vi "Teleop.vi"(10 "Match Info":T2={"Autonomous Elapsed Seconds"=0.0, "TeleOp Elapsed Seconds"=0.0, "Disabled Elapsed Seconds"=0.0, "Visited Autonomous"=FALSE, "Visited TeleOp"=FALSE, "Visited Disabled"=FALSE, "Autonomous Settings"={"Autonomous Style"=enum."Independent", "VI Refnum"=refnum}}, 11 "Call Context":T3) -> ()   [LabVIEW 2015]
doc: "This VI is called for each TeleOp packet received from the DS where the robot is not disabled. It is often used to read from the joysticks and update I/O or to update setpoints for timed control loops. It should complete and return within 20 milliseconds or it may miss DS packets."
uses:
  <vilib>/Rock Robotics/WPI/DriverStation/WPI_DriverStationDerivedRobotMode.ctl
  <vilib>/Rock Robotics/WPI/DriverStation/WPI_DriverStationMatch Info.ctl
  <vilib>/Rock Robotics/WPI/Utilities/WPI_GetSetVariantRefNum.vi
  <vilib>/Rock Robotics/Network Tables/NT Write Boolean Array.vi
  <vilib>/Rock Robotics/Network Tables/NT Write Numeric Array.vi
  <vilib>/Rock Robotics/Network Tables/NT Read Boolean.vi
  <vilib>/Rock Robotics/Network Tables/NT Read Number.vi
  Robot Global Data.vi
  <vilib>/Rock Robotics/Network Tables/NT Write Number.vi
  <vilib>/Rock Robotics/WPI/RobotDrive/WPI_RobotDriveArcadeDrive_Standard(NoSaturation).vi
panel:
  in  "Winch Lock":bool
  out "Ladder Up Start Time":u32
  in  "LadderStateMachine":i32
  out "Accelerations":T1
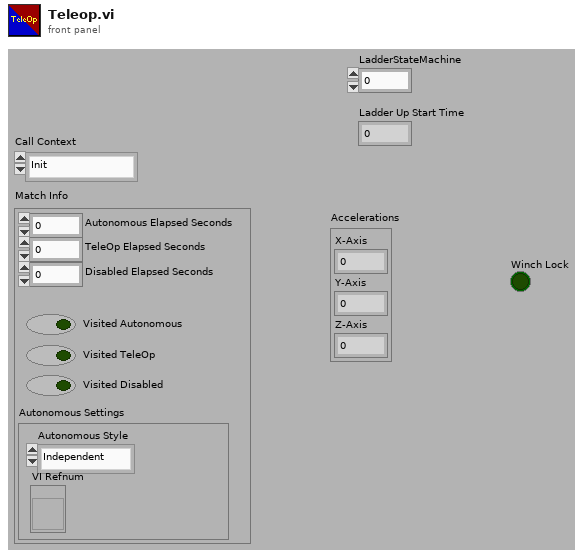
[diagram p1: front panel]
types:
  T1 = cluster{"X-Axis":dbl, "Y-Axis":dbl, "Z-Axis":dbl}
  T2 = typedef "WPI_DriverStationMatch Info.ctl" = cluster{"Autonomous Elapsed Seconds":dbl, "TeleOp Elapsed Seconds":dbl, "Disabled Elapsed Seconds":dbl, "Visited Autonomous":bool, "Visited TeleOp":bool, "Visited Disabled":bool, "Autonomous Settings":cluster{"Autonomous Style":enum16{"Iterative", "Independent"}, "VI Refnum":refnum<vi>}}
  T3 = typedef "WPI_DriverStationDerivedRobotMode.ctl" = enum16{"Init", "Execute", "Stop"}
  T4 = typedef "WPI_RobotDriveDevRef.ctl" = cluster{"DevStatus":errorcluster, "Motors[]":T5[], "Square Inputs":bool, "Max Output":dbl}
  T5 = typedef "WPI_MotorControlDeviceRef.ctl" = cluster{"DeviceStatus":errorcluster, "Type":T6, "PWM":cluster{"PWM Channel":T7, "DeadBand":T8}, "CAN":cluster{"Device Number":u8, "Control Mode":T9, "Semaphore":T10, "Max Vout":dbl, "TalonSRX Control Mode":T11}, "Invert":bool}
  T6 = typedef "WPI_MotorControlType.ctl" = enum16{"PWM", "CAN", "CANTalonSRX"}
  T7 = typedef "FPGA_DIOPWMChannel.ctl" = enum8{"PWM 0", "PWM 1", "PWM 2", "PWM 3", "PWM 4", "PWM 5", "PWM 6", "PWM 7", "PWM 8", "PWM 9", "PWM MXP 0", "PWM MXP 1", "PWM MXP 2", "PWM MXP 3", "PWM MXP 4", "PWM MXP 5", "PWM MXP 6", "PWM MXP 7", "PWM MXP 8", "PWM MXP 9", "Invalid"}
  T8 = typedef "WPI_PWMDeadband.ctl" = cluster{"Name":string, "maxPositivePwm":i32, "minPositivePwm":i32, "centerPwm":i32, "maxNegativePwm":i32, "minNegativePwm":i32, "angularRange":u16}
  T9 = typedef "WPI_CANJaguar_ControlMode.ctl" = enum8{"Percent VBus", "Current", "Speed", "Position", "Voltage"}
  T10 = typedef "Semaphore RefNum" = refnum<k1>
  T11 = typedef "WPI_CANTalonSRX_APIControlMode.ctl" = enum8{"Percent VBus", "Speed", "Position", "Slave", "Unchanged / Invalid", "Voltage Compensation", "Current", "Motion Profile"}
  T12 = typedef "WPI_JoystickDevRef.ctl" = cluster{"Device":T13}
  T13 = typedef "WPI_JoystickDeviceEnum.ctl" = enum16{"USB 0", "USB 1", "USB 2", "USB 3", "USB 4", "USB 5"}
  T14 = typedef "WPI_DigitalInputDevRef.ctl" = cluster{"DevStatus":errorcluster, "DIO Channel":T15}
  T15 = typedef "FPGA_DIOChannel.ctl" = enum8{"DIO 0", "DIO 1", "DIO 2", "DIO 3", "DIO 4", "DIO 5", "DIO 6", "DIO 7", "DIO 8", "DIO 9", "DIO MXP 0", "DIO MXP 1", "DIO MXP 2", "DIO MXP 3", "DIO MXP 4", "DIO MXP 5", "DIO MXP 6", "DIO MXP 7", "DIO MXP 8", "DIO MXP 9", "DIO MXP 10", "DIO MXP 11", "DIO MXP 12", "DIO MXP 13", "DIO MXP 14", "DIO MXP 15", "Invalid"}
  T16 = typedef "WPI_AccelerometerDevRef.ctl" = cluster{"DevStatus":errorcluster, "Scaling":T17, "Analog Channels":T18, "I2C Bus":T20, "SPI Bus":T21, "Accel Range":T22, "ADXL Axes":T23, "Handle":i32, "Device Address":u8, "Accel Type":enum16{"Analog", "ADXL345 I2C", "ADXL345 SPI", "Internal", "ADXL362 SPI"}}
  T17 = typedef "WPI_AccelerometerScaling.ctl" = cluster{"Gain (VoltsPerG)":dbl, "Center Voltage":dbl}
  T18 = typedef "WPI_AccelerometerAnalogChannels.ctl" = cluster{"X-Axis":T19, "Y-Axis":T19, "Z-Axis":T19}
  T19 = typedef "FPGA_AIChannel.ctl" = enum8{"AI 0", "AI 1", "AI 2", "AI 3", "AI MXP 0", "AI MXP 1", "AI MXP 2", "AI MXP 3", "Invalid"}
  T20 = typedef "i2c_bus.ctl" = enum16{"I2C On-Board", "I2C MXP", "Invalid"}
  T21 = typedef "spi_bus.ctl" = enum16{"SPI On-Board, CS0", "SPI On-Board, CS1", "SPI On-Board, CS2", "SPI On-Board, CS3", "SPI MXP", "Invalid"}
  T22 = typedef "ADXL345 Range.ctl" = u8
  T23 = typedef "WPI_AccelerometerADXL345 Axes.ctl" = cluster{"X-Axis":bool, "Y-Axis":bool, "Z-Axis":bool}
  T24 = typedef "WPI_EncoderDevRef.ctl" = cluster{"DevStatus":errorcluster, "EncoderIndex":T25, "CounterIndex":T26, "DistancePerCount":dbl, "Decoding Type":T27}
  T25 = typedef "FPGA_EncoderIdx.ctl" = enum8{"Enc 0", "Enc 1", "Enc 2", "Enc 3", "Enc 4", "Enc 5", "Enc 6", "Enc 7", "Invalid"}
  T26 = typedef "FPGA_CounterCtrSystemIndex.ctl" = enum8{"Ctr 0", "Ctr 1", "Ctr 2", "Ctr 3", "Ctr 4", "Ctr 5", "Ctr 6", "Ctr 7", "Invalid"}
  T27 = typedef "WPI_EncoderType.ctl" = enum16{"1x", "2x", "4x"}
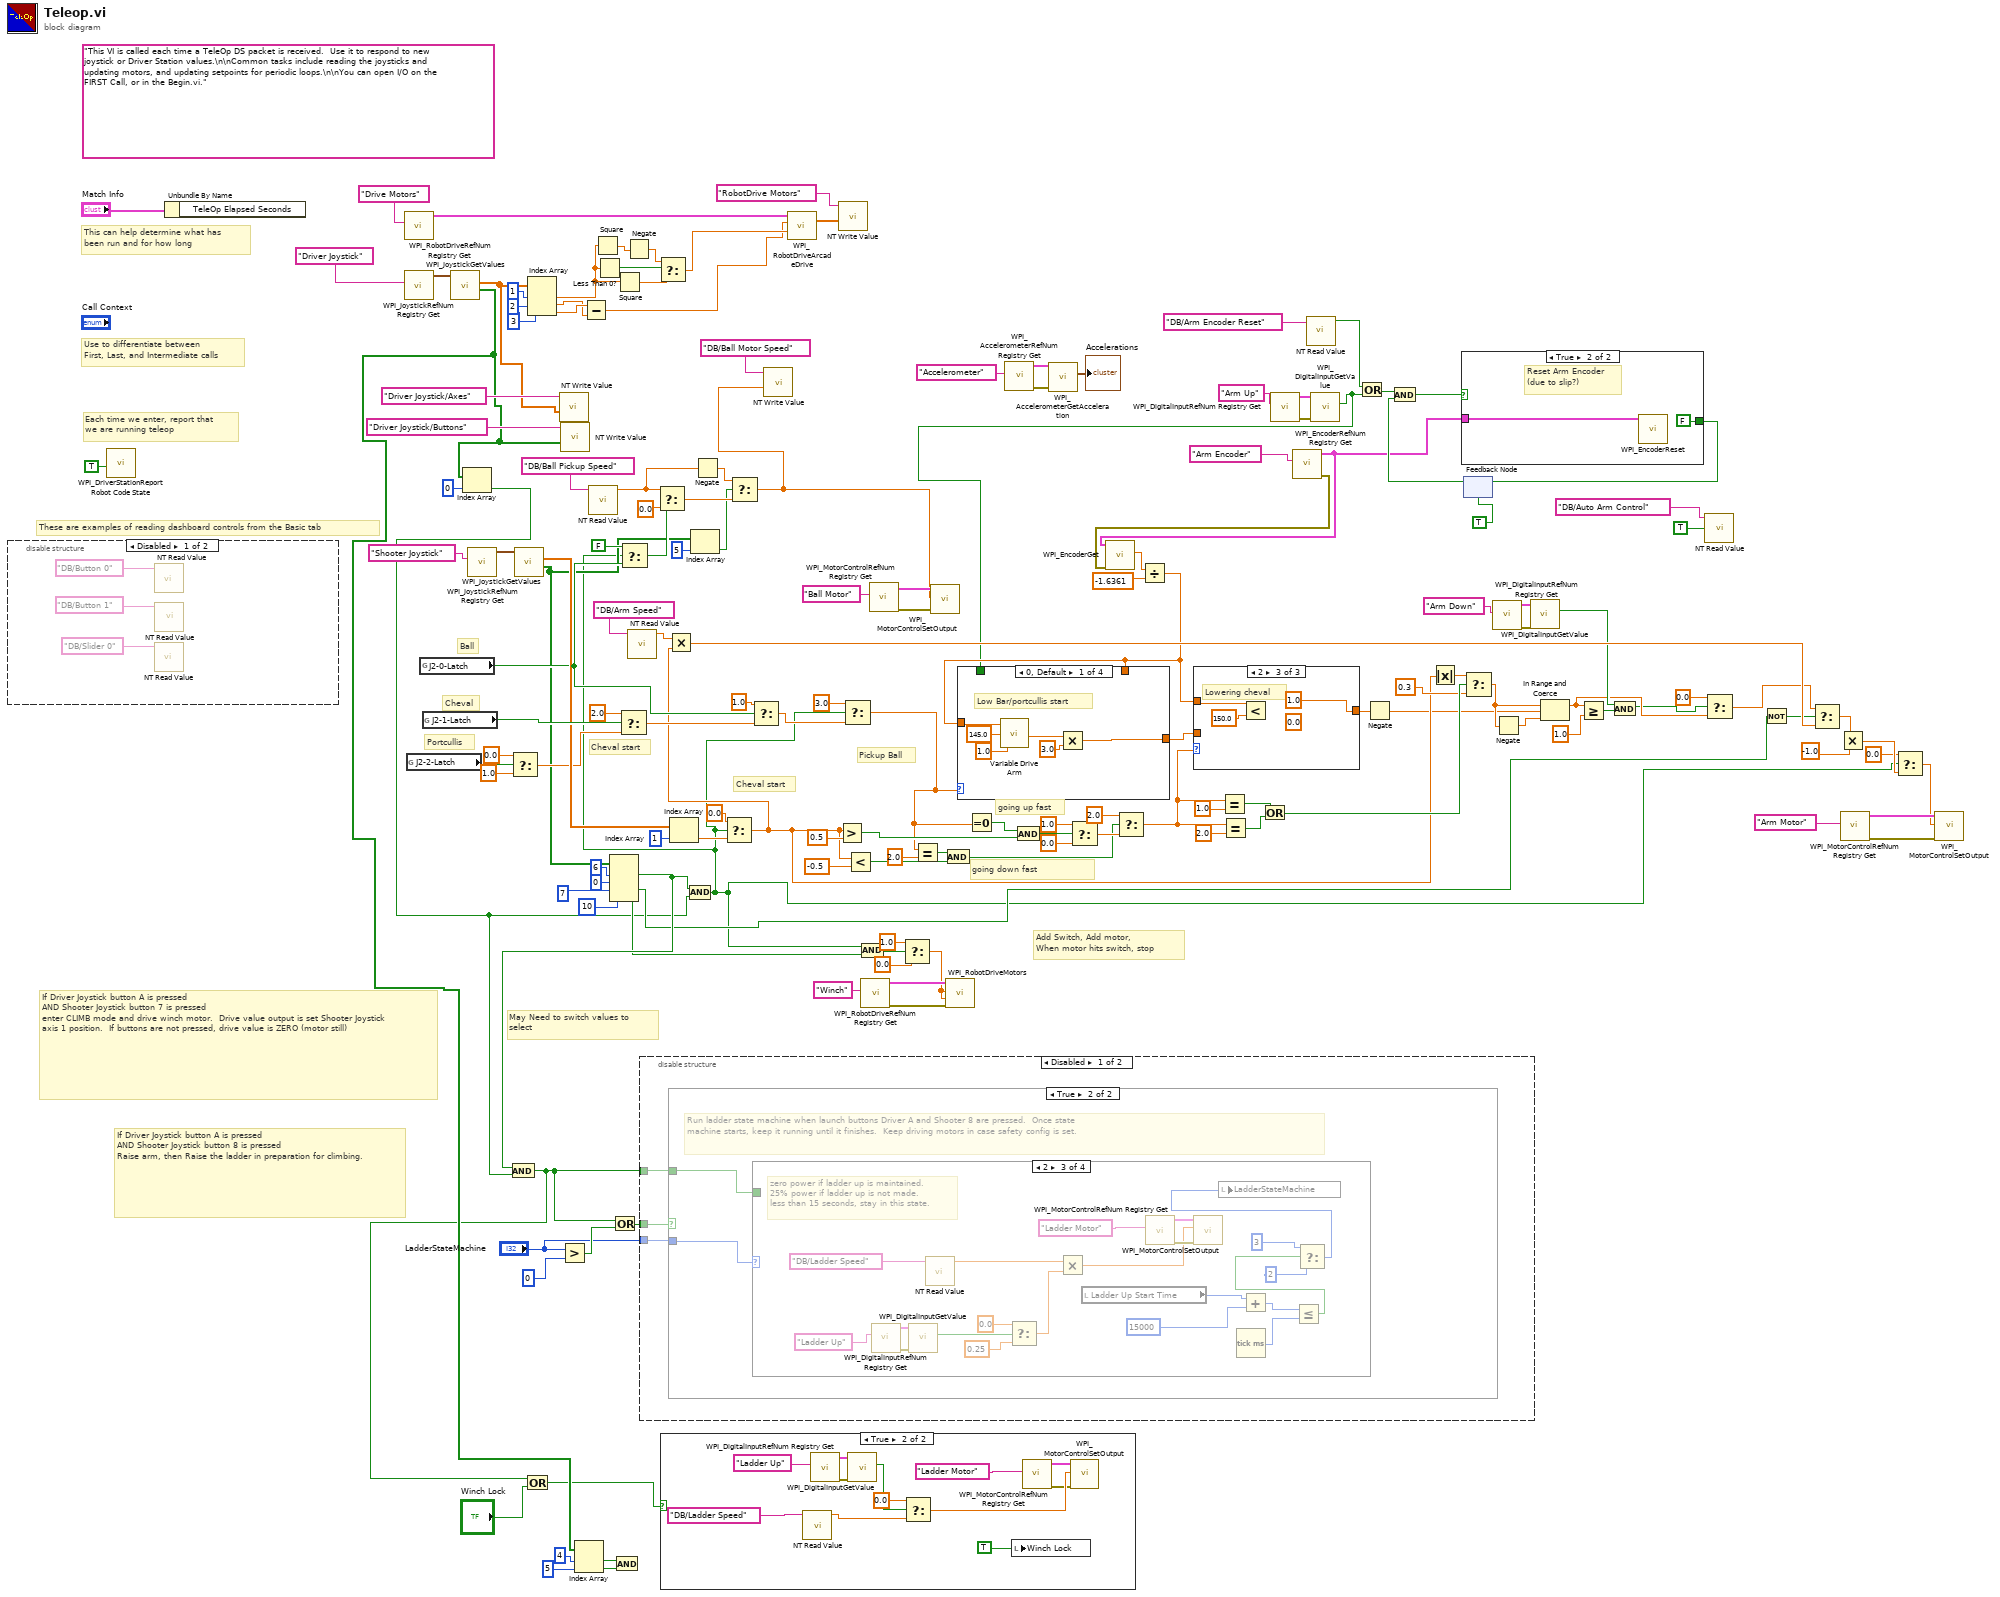
[diagram p0: block diagram]
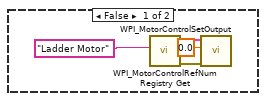
[diagram p2: hidden frame]
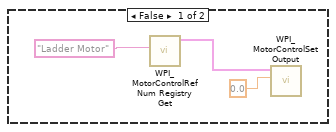
[diagram p3: hidden frame]
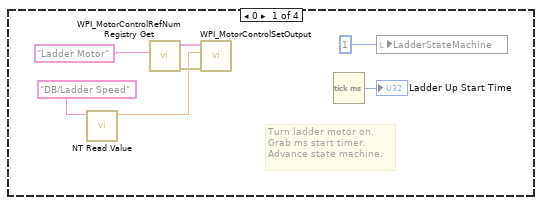
[diagram p4: hidden frame]
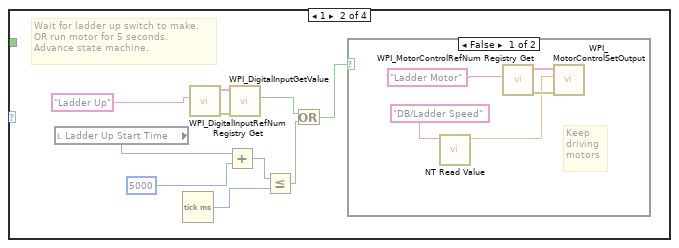
[diagram p5: hidden frame]
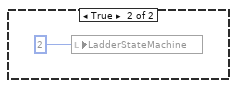
[diagram p6: hidden frame]
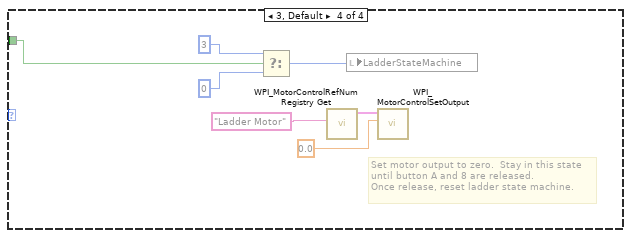
[diagram p7: hidden frame]
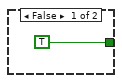
[diagram p9: hidden frame]
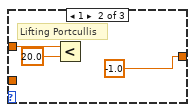
[diagram p12: hidden frame]
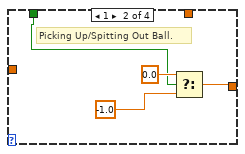
[diagram p13: hidden frame]
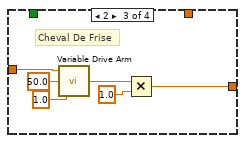
[diagram p14: hidden frame]
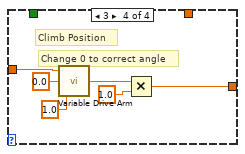
[diagram p15: hidden frame]
diagram:
  (unwired) "This VI is called each time a TeleOp DS packet is received.  Use it to respond to new joystick or Driver Station values.\n\nCommon tasks include reading the joysticks and updating motors, and updating setpoints for periodic loops.\n\nYou can open I/O on the FIRST Call, or in the Begin.vi."
  # "going up fast"
  # "going down fast"
  # "If Driver Joystick button A is pressed\nAND Shooter Joystick button 8 is pressed\nRaise arm, then Raise the ladder in preparation for climbing."
  # "If Driver Joystick button A is pressed\nAND Shooter Joystick button 7 is pressed\nenter CLIMB mode and drive winch motor.  Drive value output is set Shooter Joystick axis 1 position.  If buttons are not pressed, drive value is ZERO (motor still)"
  # "Add Switch, Add motor, \nWhen motor hits switch, stop"
  # "Portcullis"
  # "Ball"
  # "Cheval"
  # "May Need to switch values to \nselect"
  # "Cheval start"
  # "Pickup Ball"
  # "Cheval start"
  # "These are examples of reading dashboard controls from the Basic tab"
  # "Each time we enter, report that\nwe are running teleop"
  # "Use to differentiate between\nFirst, Last, and Intermediate calls"
  # "This can help determine what has\nbeen run and for how long"
  n1 = disable-structure shown="Disabled" {
    frame Disabled {
      n2 = call-poly <vilib>:"NT Read Value.vi"("Name"="DB/Button 0" ("refnum name")) -> ("Boolean"=w158:bool)  [unwired: 9 in, 1 out]
      n3 = call-poly <vilib>:"NT Read Value.vi"("Name"="DB/Slider 0" ("refnum name")) -> ("Numeric"=w160:dbl)  [unwired: 9 in, 1 out]
      n4 = call-poly <vilib>:"NT Read Value.vi"("Name"="DB/Button 1" ("refnum name")) -> ("Boolean"=w159:bool)  [unwired: 9 in, 1 out]
    }
    frame Enabled {
    }
  }
  n5 = call <vilib>:"WPI_DriverStationReport Robot Code State.vi"("TeleOp"=TRUE ("Autonomous")) -> ()  [unwired: 10 in, 1 out]
  n6 = Unbundle By Name("Match Info") -> ()  [unwired: 1 out]
  n7 = call <vilib>:"WPI_RobotDriveRefNum Registry Get.vi"("refnum name"="Drive Motors") -> ("RobotDriveDevRef"=w154:T4)  [unwired: 1 in, 9 out]
  n8 = call <vilib>:"WPI_JoystickRefNum Registry Get.vi"("refnum name"="Driver Joystick") -> ("JoystickDevRef"=w152:T12)  [unwired: 1 in, 9 out]
  n9 = global read "Robot Global Data.vi" "J2-2-Latch"() -> (w77:bool)
  n10 = global read "Robot Global Data.vi" "J2-0-Latch"() -> (w73:bool)
  n11 = global read "Robot Global Data.vi" "J2-1-Latch"() -> (w130:bool)
  n12 = call <vilib>:"WPI_JoystickGetValues.vi"("JoystickDevRef"=w152) -> ("Buttons"=w20:bool[], "Axes"=w142:dbl[])  [unwired: 6 in, 3 out]
  n13 = Index Array(array=w20, index=0) -> (element=w19:bool)
  n14 = call <vilib>:"WPI_JoystickRefNum Registry Get.vi"("refnum name"="Shooter Joystick") -> ("JoystickDevRef"=w141:T12)  [unwired: 1 in, 9 out]
  n15 = Select(t=0.0, s=w77, f=1.0) -> (s? t:f=w78:dbl)
  n16 = call <vilib>:"WPI_JoystickGetValues.vi"("JoystickDevRef"=w141) -> ("Buttons"=w44:bool[], "Axes"=w106:dbl[])  [unwired: 6 in, 3 out]
  n17 = Index Array(array=w142, index #1=1 ("index"), index #2=2 ("index"), index #3=3 ("index")) -> (element #1=w102:dbl, element #2=w99:dbl, element #3=w100:dbl)
  n18 = call-poly <vilib>:"NT Write Value.vi"("Numeric Array"=w142, "Name"="Driver Joystick/Axes") -> ()  [unwired: 9 in, 1 out]
  n19 = call-poly <vilib>:"NT Write Value.vi"("Boolean Array"=w20, "Name"="Driver Joystick/Buttons") -> ()  [unwired: 9 in, 1 out]
  n20 = Greater?(x="LadderStateMachine", y=0) -> (0:w58:bool)
  n21 = Index Array(array=w20, index #1=4 ("index"), index #2=5 ("index")) -> (element #1=w15:bool, element #2=w16:bool)
  n22 = Subtract(x=w100, y=w99) -> (x-y=w98:dbl)
  n23 = call-poly <vilib>:"NT Read Value.vi"("Name"="DB/Ball Pickup Speed") -> ("Numeric"=w45:dbl)  [unwired: 9 in, 1 out]
  n24 = Square(x=w102) -> (x^2=w146:dbl)
  n25 = Less Than 0?(x=w102) -> (x < 0?=w148:bool)
  n26 = Index Array(array=w44, index #1=6 ("index"), index #2=0 ("index"), index #3=7 ("index"), index #4=10 ("index")) -> (element #1=w55:bool, element #3=w36:bool, element #4=w24:bool)  [unwired: 1 out]
  n27 = And(x=w55, y=w19) -> (x .and. y?=w13:bool)
  n28 = Or(x=w13, y="Winch Lock") -> (x .or. y?=w2:bool)
  n29 = Or(x=w13, y=w58) -> (x .or. y?=w57:bool)
  n30 = And(x=w15, y=w16) -> ()  [unwired: 1 out]
  n31 = Square(x=w102) -> (x^2=w145:dbl)
  n32 = Select(t=2.0, s=w130, f=w78) -> (s? t:f=w131:dbl)
  n33 = Negate(x=w146) -> (-x=w147:dbl)
  n34 = call-poly <vilib>:"NT Read Value.vi"("Name"="DB/Arm Speed") -> ("Numeric"=w67:dbl)  [unwired: 9 in, 1 out]
  n35 = disable-structure shown="Disabled" {
    disable-tunnel: w57 -> [w166 _]
    disable-tunnel: "LadderStateMachine" -> [w165 _]
    disable-tunnel: w13 -> [w164 _]
    frame Disabled {
      n36 = case shown="True" w166 {
        tunnel: w165 -> [_ w171]
        tunnel: w164 -> [_ w170]
        frame False {
          n37 = call <vilib>:"WPI_MotorControlRefNum Registry Get.vi"("refnum name"="Ladder Motor") -> ("MotorControlDevRef"=w167:T5)  [unwired: 9 in, 1 out]
          n38 = call <vilib>:"WPI_MotorControlSetOutput.vi"("Output"=0.0, "MotorControlDevRef"=w167) -> ()  [unwired: 7 in, 3 out]
        }
        frame True {
          # "Run ladder state machine when launch buttons Driver A and Shooter 8 are pressed.  Once state\nmachine starts, keep it running until it finishes.  Keep driving motors in case safety config is set."
          n39 = case shown="2" w171 {
            tunnel: w170 -> [_ _ _ w220]
            frame 0 {
              # "Turn ladder motor on.\nGrab ms start timer.\nAdvance state machine."
              n40 = call-poly <vilib>:"NT Read Value.vi"("Name"="DB/Ladder Speed") -> ("Numeric"=w174:dbl)  [unwired: 9 in, 1 out]
              n41 = call <vilib>:"WPI_MotorControlRefNum Registry Get.vi"("refnum name"="Ladder Motor") -> ("error out"=w178:errorcluster, "MotorControlDevRef"=w177:T5)  [unwired: 9 in]
              n42 = call <vilib>:"WPI_MotorControlSetOutput.vi"("error in (no error)"=w178, "Output"=w174, "MotorControlDevRef"=w177) -> ()  [unwired: 6 in, 3 out]
              n43 = Tick Count (ms)() -> (millisecond timer value=→"Ladder Up Start Time":u32)
              n44 = local write "LadderStateMachine"(1 ("LadderStateMachine")) -> ()
            }
            frame 1 {
              # "Wait for ladder up switch to make.\nOR run motor for 5 seconds.\nAdvance state machine."
              n45 = local read "Ladder Up Start Time"() -> (w184:u32)
              n46 = Tick Count (ms)() -> (millisecond timer value=w182:u32)
              n47 = call <vilib>:"WPI_DigitalInputRefNum Registry Get.vi"("refnum name"="Ladder Up") -> ("error out"=w188:errorcluster, "DigitalInputDevRef"=w186:T14)  [unwired: 9 in]
              n48 = Add(x=w184, y=u32 5000) -> (x+y=w183:u32)
              n49 = call <vilib>:"WPI_DigitalInputGetValue.vi"("error in (no error)"=w188, "DigitalInputDevRef"=w186) -> ("Value"=w179:bool)  [unwired: 7 in, 2 out]
              n50 = Less Or Equal?(x=w183, y=w182) -> (x <= y?=w180:bool)
              n51 = Or(x=w179, y=w180) -> (x .or. y?=w181:bool)
              n52 = case shown="False" w181 {
                frame False {
                  # "Keep\ndriving \nmotors"
                  n53 = call-poly <vilib>:"NT Read Value.vi"("Name"="DB/Ladder Speed") -> ("Numeric"=w189:dbl)  [unwired: 9 in, 1 out]
                  n54 = call <vilib>:"WPI_MotorControlRefNum Registry Get.vi"("refnum name"="Ladder Motor") -> ("error out"=w193:errorcluster, "MotorControlDevRef"=w192:T5)  [unwired: 9 in]
                  n55 = call <vilib>:"WPI_MotorControlSetOutput.vi"("error in (no error)"=w193, "Output"=w189, "MotorControlDevRef"=w192) -> ()  [unwired: 6 in, 3 out]
                }
                frame True {
                  n56 = local write "LadderStateMachine"(2 ("LadderStateMachine")) -> ()
                }
              }
            }
            frame 2 {
              # "zero power if ladder up is maintained.\n25% power if ladder up is not made.\nless than 15 seconds, stay in this state."
              n57 = call <vilib>:"WPI_DigitalInputRefNum Registry Get.vi"("refnum name"="Ladder Up") -> ("error out"=w209:errorcluster, "DigitalInputDevRef"=w207:T14)  [unwired: 9 in]
              n58 = call <vilib>:"WPI_DigitalInputGetValue.vi"("error in (no error)"=w209, "DigitalInputDevRef"=w207) -> ("Value"=w206:bool)  [unwired: 7 in, 2 out]
              n59 = call-poly <vilib>:"NT Read Value.vi"("Name"="DB/Ladder Speed") -> ("Numeric"=w211:dbl)  [unwired: 9 in, 1 out]
              n60 = Select(t=0.0, s=w206, f=0.25 ("y")) -> (s? t:f=w203:dbl)
              n61 = Multiply(x=w211, y=w203) -> (x*y=w210:dbl)
              n62 = local read "Ladder Up Start Time"() -> (w201:u32)
              n63 = call <vilib>:"WPI_MotorControlRefNum Registry Get.vi"("refnum name"="Ladder Motor") -> ("error out"=w215:errorcluster, "MotorControlDevRef"=w214:T5)  [unwired: 9 in]
              n64 = call <vilib>:"WPI_MotorControlSetOutput.vi"("error in (no error)"=w215, "Output"=w210, "MotorControlDevRef"=w214) -> ()  [unwired: 6 in, 3 out]
              n65 = Tick Count (ms)() -> (millisecond timer value=w199:u32)
              n66 = Add(x=w201, y=u32 15000) -> (x+y=w200:u32)
              n67 = Less Or Equal?(x=w200, y=w199) -> (x <= y?=w198:bool)
              n68 = Select(t=3 ("LadderStateMachine"), s=w198, f=2) -> (s? t:f=w195:i32)
              n69 = local write "LadderStateMachine"(w195) -> ()
            }
            frame 3, Default {
              # "Set motor output to zero.  Stay in this state\nuntil button A and 8 are released.\nOnce release, reset ladder state machine."
              n70 = Select(t=3 ("y"), s=w220, f=0 ("y")) -> (s? t:f=w219:i32)
              n71 = call <vilib>:"WPI_MotorControlRefNum Registry Get.vi"("refnum name"="Ladder Motor") -> ("MotorControlDevRef"=w218:T5)  [unwired: 9 in, 1 out]
              n72 = local write "LadderStateMachine"(w219) -> ()
              n73 = call <vilib>:"WPI_MotorControlSetOutput.vi"("Output"=0.0, "MotorControlDevRef"=w218) -> ()  [unwired: 7 in, 3 out]
            }
          }
        }
      }
    }
    frame Enabled {
    }
  }
  n74 = Select(t=w147, s=w148, f=w145) -> (s? t:f=w105:dbl)
  n75 = case shown="True" w2 {
    frame False {
      n76 = call <vilib>:"WPI_MotorControlRefNum Registry Get.vi"("refnum name"="Ladder Motor") -> ("error out"=w224:errorcluster, "MotorControlDevRef"=w226:T5)  [unwired: 9 in]
      n77 = call <vilib>:"WPI_MotorControlSetOutput.vi"("error in (no error)"=w224, "Output"=0.0, "MotorControlDevRef"=w226) -> ()  [unwired: 6 in, 3 out]
    }
    frame True {
      n78 = call-poly <vilib>:"NT Read Value.vi"("Name"="DB/Ladder Speed") -> ("Numeric"=w232:dbl)  [unwired: 9 in, 1 out]
      n79 = call <vilib>:"WPI_DigitalInputRefNum Registry Get.vi"("refnum name"="Ladder Up") -> ("error out"=w238:errorcluster, "DigitalInputDevRef"=w236:T14)  [unwired: 9 in]
      n80 = call <vilib>:"WPI_DigitalInputGetValue.vi"("error in (no error)"=w238, "DigitalInputDevRef"=w236) -> ("Value"=w235:bool)  [unwired: 7 in, 2 out]
      n81 = Select(t=0.0, s=w235, f=w232) -> (s? t:f=w229:dbl)
      n82 = local write "Winch Lock"(TRUE) -> ()
      n83 = call <vilib>:"WPI_MotorControlRefNum Registry Get.vi"("refnum name"="Ladder Motor") -> ("error out"=w228:errorcluster, "MotorControlDevRef"=w231:T5)  [unwired: 9 in]
      n84 = call <vilib>:"WPI_MotorControlSetOutput.vi"("error in (no error)"=w228, "Output"=w229, "MotorControlDevRef"=w231) -> ()  [unwired: 6 in, 3 out]
    }
  }
  n85 = Index Array(array=w106, index=1) -> (element=w97:dbl)
  n86 = And(x=w55, y=w19) -> (x .and. y?=w26:bool)
  n87 = Select(t=FALSE, s=w26, f=w73) -> (s? t:f=w74:bool)
  n88 = Select(t=w45, s=w74, f=0.0) -> (s? t:f=w47:dbl)
  n89 = Index Array(array=w44, index=5) -> (element=w42:bool)
  n90 = Negate(x=w45) -> (-x=w46:dbl)
  n91 = Select(t=0.0, s=w26, f=w97) -> (s? t:f=w68:dbl)
  n92 = Multiply(x=w67, y=w68) -> (x*y=w63:dbl)
  n93 = Select(t=w46, s=w42, f=w47) -> (s? t:f=w1:dbl)
  n94 = Select(t=1.0, s=w73, f=w131) -> (s? t:f=w82:dbl)
  n95 = call-poly <vilib>:"NT Write Value.vi"("Numeric"=w1, "Name"="DB/Ball Motor Speed") -> ()  [unwired: 9 in, 1 out]
  n96 = call-poly <vilib>:"WPI_RobotDriveArcadeDrive.vi"("Y axis value"=w105, "X axis value"=w98, "RobotDriveDevRef"=w154) -> ("Motor Values"=w151:dbl[])  [unwired: 6 in, 2 out]
  n97 = Greater?(x=w68, y=0.5) -> (0:w126:bool)
  n98 = call-poly <vilib>:"NT Write Value.vi"("Numeric Array"=w151, "Name"="RobotDrive Motors") -> ()  [unwired: 9 in, 1 out]
  n99 = Select(t=3.0, s=w26, f=w82) -> (s? t:f=w83:dbl)
  n100 = Less?(x=w68, y=-0.5) -> (x < y?=w120:bool)
  n101 = And(x=w26, y=w24) -> (x .and. y?=w27:bool)
  n102 = call <vilib>:"WPI_RobotDriveRefNum Registry Get.vi"("refnum name"="Winch") -> ("error out"=w112:errorcluster, "RobotDriveDevRef"=w111:T4)  [unwired: 9 in]
  n103 = call <vilib>:"WPI_MotorControlRefNum Registry Get.vi"("refnum name"="Ball Motor") -> ("error out"=w134:errorcluster, "MotorControlDevRef"=w135:T5)  [unwired: 9 in]
  n104 = Select(t=1.0, s=w27, f=0.0) -> (s? t:f=w28:dbl)
  n105 = Equal?(x=w83, y=2.0) -> (x = y?=w119:bool)
  n106 = call <vilib>:"WPI_MotorControlSetOutput.vi"("error in (no error)"=w134, "Output"=w1, "MotorControlDevRef"=w135) -> ()  [unwired: 6 in, 3 out]
  n107 = And(x=w119, y=w120) -> (x .and. y?=w116:bool)
  n108 = call <vilib>:"WPI_RobotDriveMotors.vi"("error in (no error)"=w112, "RightSpeed"=w28, "LeftSpeed"=w28, "RobotDriveDevRef"=w111) -> ()  [unwired: 5 in, 3 out]
  n109 = Equal To 0?(x=w83) -> (x = 0?=w129:bool)
  n110 = call <vilib>:"WPI_AccelerometerRefNum Registry Get.vi"("refnum name"="Accelerometer") -> ("error out"=w109:errorcluster, "AccelerometerDevRef"=w108:T16)  [unwired: 9 in]
  n111 = And(x=w129, y=w126) -> (x .and. y?=w125:bool)
  n112 = call <vilib>:"WPI_AccelerometerGetAcceleration.vi"("error in"=w109, "AccelerometerDevRef"=w108) -> ("Accelerations"=→"Accelerations":T1)  [unwired: 7 in, 2 out]
  n113 = Select(t=1.0, s=w125, f=0.0) -> (s? t:f=w117:dbl)
  n114 = Select(t=2.0, s=w116, f=w117) -> (s? t:f=w94:dbl)
  n115 = Equal?(x=w94, y=1.0) -> (x = y?=w92:bool)
  n116 = Equal?(x=w94, y=2.0) -> (x = y?=w91:bool)
  n117 = Or(x=w92, y=w91) -> (x .or. y?=w90:bool)
  n118 = call <vilib>:"WPI_DigitalInputRefNum Registry Get.vi"("refnum name"="Arm Up") -> ("error out"=w31:errorcluster, "DigitalInputDevRef"=w30:T14)  [unwired: 9 in]
  n119 = call <vilib>:"WPI_EncoderRefNum Registry Get.vi"("refnum name"="Arm Encoder") -> ("error out"=w52:errorcluster, "EncoderDevRef"=w53:T24)  [unwired: 9 in]
  n120 = call <vilib>:"WPI_EncoderGet.vi"("error in (no error)"=w52, "EncoderDevRef"=w53) -> ("Distance"=w50:dbl)  [unwired: 4 in, 5 out]
  n121 = Divide(x=w50, y=-1.6361 ("Arm Calibration")) -> (x/y=w49:dbl)
  n122 = call-poly <vilib>:"NT Read Value.vi"("Name"="DB/Arm Encoder Reset") -> ("Boolean"=w33:bool)  [unwired: 9 in, 1 out]
  n123 = call <vilib>:"WPI_DigitalInputGetValue.vi"("error in (no error)"=w31, "DigitalInputDevRef"=w30) -> ("Value"=w29:bool)  [unwired: 7 in, 2 out]
  n124 = case shown="0, Default" w83 {
    tunnel: w49 -> [w244 _ w249 w255]
    tunnel: [w241 w248 w250 w256] -> w122
    tunnel: w49 -> [_ _ _ _]
    tunnel: w29 -> [_ w245 _ _]
    frame 0, Default {
      # "Low Bar/portcullis start"
      n125 = call "Variable Drive Arm.vi"("Max Speed"=1.0, "Wanted Angle"=145.0, "Encoder"=w244) -> ("Motor Controller"=w240:dbl)
      n126 = Multiply(x=w240, y=3.0) -> (x*y=w241:dbl)
    }
    frame 1 {
      # "Picking Up/Spitting Out Ball."
      n127 = Select(t=0.0, s=w245, f=-1.0) -> (s? t:f=w248:dbl)
    }
    frame 2 {
      # "Cheval De Frise"
      n128 = call "Variable Drive Arm.vi"("Max Speed"=1.0, "Wanted Angle"=50.0, "Encoder"=w249) -> ("Motor Controller"=w252:dbl)
      n129 = Multiply(x=w252, y=1.0) -> (x*y=w250:dbl)
    }
    frame 3 {
      # "Change 0 to correct angle"
      # "Climb Position"
      n130 = call "Variable Drive Arm.vi"("Max Speed"=1.0, "Wanted Angle"=0.0, "Encoder"=w255) -> ("Motor Controller"=w258:dbl)
      n131 = Multiply(x=w258, y=1.0) -> (x*y=w256:dbl)
    }
  }
  n132 = case shown="2" w94 {
    tunnel: w49 -> [_ w264 w267]
    tunnel: [w261 -1.0 ("f") 1.0 ("t")] -> w86
    tunnel: w122 -> [w261 _ _]
    frame 0, Default {
    }
    frame 1 {
      # "Lifting Portcullis"
      n133 = Less?(x=w264, y=20.0) -> ()  [unwired: 1 out]
    }
    frame 2 {
      (unwired) 0.0 ("f")
      # "Lowering cheval"
      n134 = Less?(x=w267, y=150.0) -> ()  [unwired: 1 out]
    }
  }
  n135 = Or(x=w33, y=w29) -> (x .or. y?=w34:bool)
  n136 = Negate(x=w86) -> (-x=w41:dbl)
  n137 = Absolute Value(x=w68) -> (abs(x)=w89:dbl)
  n138 = feedback #1(TRUE) -> (w61:bool)
  n139 = And(x=w34, y=w61) -> (x .and. y?=w48:bool)
  n140 = case shown="True" w48 {
    tunnel: [TRUE FALSE] -> w60
    tunnel: w53 -> [_ w269]
    frame False {
    }
    frame True {
      # "Reset Arm Encoder\n(due to slip?)"
      n141 = call <vilib>:"WPI_EncoderReset.vi"("EncoderDevRef"=w269) -> ()  [unwired: 9 in, 2 out]
    }
  }
  n142 = feedback-in #1(w60) -> ()
  n143 = Select(t=w89, s=w90, f=0.3) -> (s? t:f=w87:dbl)
  n144 = call <vilib>:"WPI_DigitalInputRefNum Registry Get.vi"("refnum name"="Arm Down") -> ("error out"=w10:errorcluster, "DigitalInputDevRef"=w9:T14)  [unwired: 9 in]
  n145 = Negate(x=w87) -> (-x=w88:dbl)
  n146 = call <vilib>:"WPI_DigitalInputGetValue.vi"("error in (no error)"=w10, "DigitalInputDevRef"=w9) -> ("Value"=w7:bool)  [unwired: 7 in, 2 out]
  n147 = In Range and Coerce(upper limit=w87, x=w41, lower limit=w88) -> (coerced(x)=w5:dbl)  [unwired: 1 out]
  n148 = Greater Or Equal?(x=w5, y=1.0 ("x")) -> (x >= y?=w11:bool)
  n149 = And(x=w7, y=w11) -> (x .and. y?=w3:bool)
  n150 = call-poly <vilib>:"NT Read Value.vi"("Default Value"=TRUE, "Name"="DB/Auto Arm Control") -> ()  [unwired: 8 in, 2 out]
  n151 = Select(t=0.0, s=w3, f=w5) -> (s? t:f=w6:dbl)
  n152 = Not(x=w36) -> (.not. x?=w35:bool)
  n153 = Select(t=w6, s=w35, f=w63) -> (s? t:f=w96:dbl)
  n154 = Multiply(x=w96, y=-1.0) -> (x*y=w39:dbl)
  n155 = call <vilib>:"WPI_MotorControlRefNum Registry Get.vi"("refnum name"="Arm Motor") -> ("error out"=w137:errorcluster, "MotorControlDevRef"=w138:T5)  [unwired: 9 in]
  n156 = Select(t=0.0, s=w26, f=w39) -> (s? t:f=w40:dbl)
  n157 = call <vilib>:"WPI_MotorControlSetOutput.vi"("error in (no error)"=w137, "Output"=w40, "MotorControlDevRef"=w138) -> ()  [unwired: 6 in, 3 out]
